vi "Reaction Wheel PID.vi"(2 "PID output range":cluster{"Maximum":dbl, "Minimum":dbl}, 3 "PID gains":cluster{"P":dbl, "I":dbl, "D":dbl}, 4 "Roll":dbl, 5 "Roll reference":dbl) -> (0 "PID output":dbl)   [LabVIEW 2021]
uses:
  <vilib>/addons/control/pid/pid.llb/PID (DBL).vi
  <vilib>/addons/control/pid/NI_PID_pid.lvlib
panel:
  # "Roll reference should be zero wheen reaction \nwheel is used, i.e. when the bike is standing still."
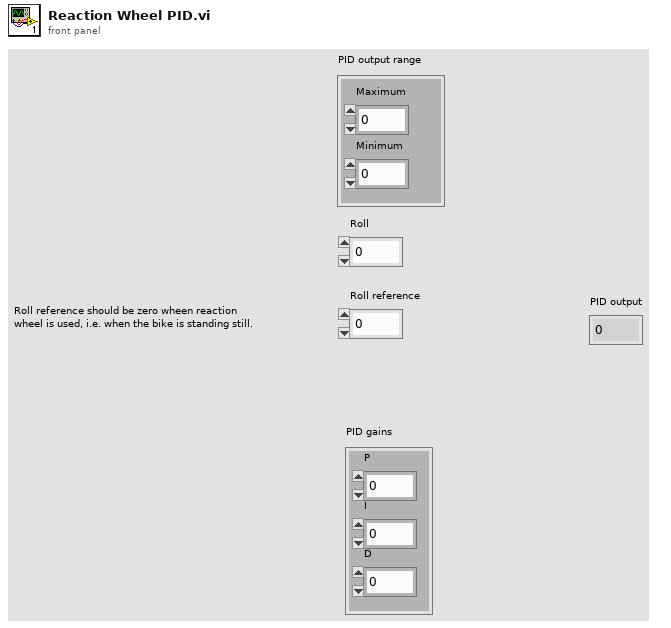
[diagram p1: front panel]
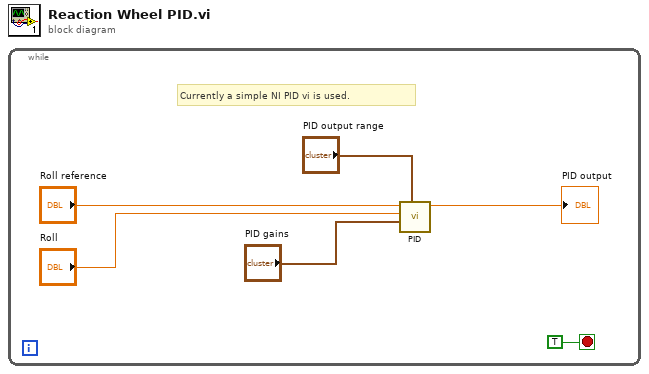
[diagram p0: block diagram]
diagram:
  n1 = while {
    stop <- TRUE stop-if-true
    # "Currently a simple NI PID vi is used."
    n2 = call-poly <vilib>:"PID.vi"("output range"="PID output range", "PID gains"="PID gains", "process variable"="Roll", "setpoint"="Roll reference") -> ("output"=→"PID output":dbl)  [unwired: 6 in, 1 out]
  }
